vi "save_config_file.vi"(8 "error in (no error)":errorcluster, 11 "GenericPlugin in":refnum<class "GenericComponent.lvclass">) -> (0 "error out":errorcluster, 3 "GenericPlugin out":refnum<class "GenericComponent.lvclass">)   [LabVIEW 2010, in "GenericComponent.lvclass"]
uses:
  GenericComponent.lvclass
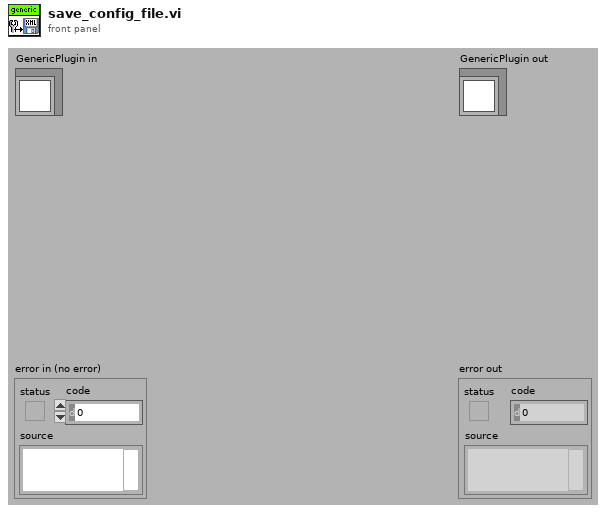
[diagram p1: front panel]
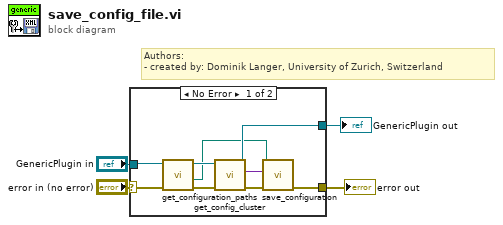
[diagram p0: block diagram]
diagram:
  # "Authors: \n- created by: Dominik Langer, University of Zurich, Switzerland"
  n1 = case shown="No Error" "error in (no error)" {
    selector: "error in (no error)" -> [w9 w15]
    tunnel: [w13 w15] -> w3
    tunnel: [w12 w14] -> w1
    tunnel: "GenericPlugin in" -> [w8 w14]
    frame No Error {
      n2 = call-dynamic "get_configuration_paths.vi"("error in (no error)"=w9, "GenericComponent in"=w8) -> ("error out"=w7:errorcluster, "configuration file path"=w5:path, "GenericComponent out"=w6:refnum<class "GenericComponent.lvclass">)  [unwired: 2 in, 5 out]
      n3 = call-dynamic "get_config_cluster.vi"("error in (no error)"=w7, "GenericComponent in"=w6) -> ("error out"=w10:errorcluster, "config cluster (variant)"=w11:variant, "GenericComponent out"=w12:refnum<class "GenericComponent.lvclass">)  [unwired: 7 in]
      n4 = call "save_configuration.vi"("error in (no error)"=w10, "config cluster variant in (data type)"=w11, "path"=w5) -> ("error out"=w13:errorcluster)  [unwired: 4 in, 4 out]
    }
    frame Error {
    }
  }
  "error out" <- w3
  "GenericPlugin out" <- w1
